vi "macro_vecBuilder6x1FIll.vi"   [LabVIEW 2019, in "Trajectory_Library.lvlib"]
uses:
  Trajectory_Library.lvlib
  MatBuilder_Create.vi
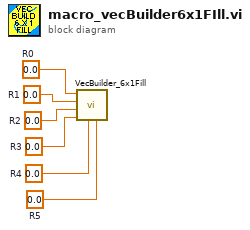
[diagram p0: block diagram]
diagram:
  w1 = 0.0  # R5
  w2 = 0.0  # R4
  w3 = 0.0  # R3
  w4 = 0.0  # R2
  w5 = 0.0  # R1
  w6 = 0.0  # R0
  n1 = call "VecBuilder_6x1Fill.vi"("R5"=w1, "R4"=w2, "R3"=w3, "R2"=w4, "R1"=w5, "R0"=w6) -> ()  [unwired: 5 in, 1 out]
